vi "PID.vi"() -> ()   [LabVIEW 2019]
panel:
  in  "PID":T1
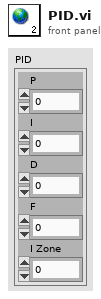
[diagram p1: front panel]
types:
  T1 = cluster{"P":dbl, "I":dbl, "D":dbl, "F":dbl, "I Zone":dbl}
diagram:
